vi "Initialize Hardware.vi"(7 "hardware config file":path, 8 "error in":errorcluster, 11 "device parameters":T2) -> (0 "error out":errorcluster, 3 "hardware handles":T1)   [LabVIEW 2020, in "Ballard MIL-STD-1553 Engine.lvlib" / "Custom Device.lvlib"]
uses:
  Custom Device.lvlib
  <instrlib>/BTICardLib/BTICardLV.lvlib
  <instrlib>/BTICardLib/Private/IO/Action-Status/Write External LED.vi
  <instrlib>/BTI1553Lib/BTI1553LV.lvlib
  Hardware Handles.ctl
  <instrlib>/BTI1553Lib/Private/Channel/Configure/Configure All From XML.vi
  <instrlib>/BTICardLib/Private/Initialize By Slot Number and Core Number.vi
  <instrlib>/BTICardLib/Private/Initialize By Card Number and Core Number.vi
  Shared/Device Parameters.ctl
  Shared/Initialization Method.ctl
panel:
  out "type string out":string
  out "product string out":string
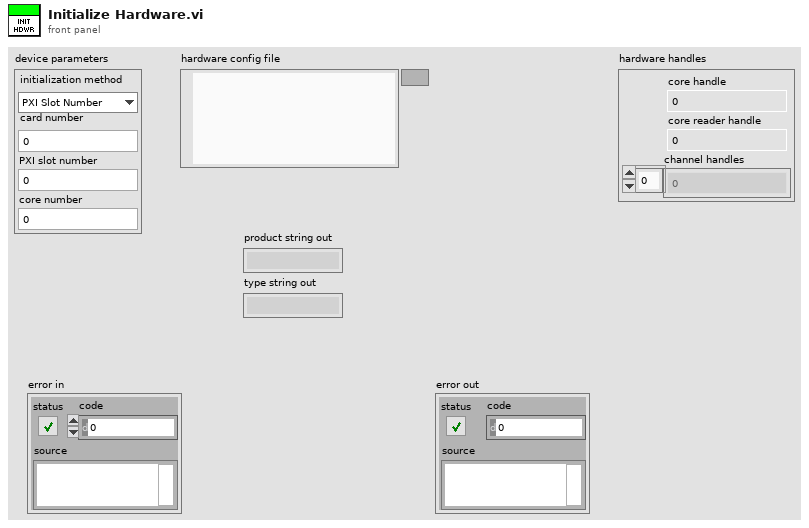
[diagram p1: front panel]
types:
  T1 = typedef "Ballard MIL-STD-1553 Engine.lvlib/Custom Device.lvlib/Hardware Handles.ctl" = cluster{"core handle":u64, "core reader handle":u64, "channel handles":u64[]}
  T2 = typedef "Device Parameters.ctl" = cluster{"initialization method":T3, "card number":i32, "PXI slot number":i32, "core number":i32}
  T3 = typedef "Initialization Method.ctl" = enum16{"PXI Slot Number", "Card Number"}
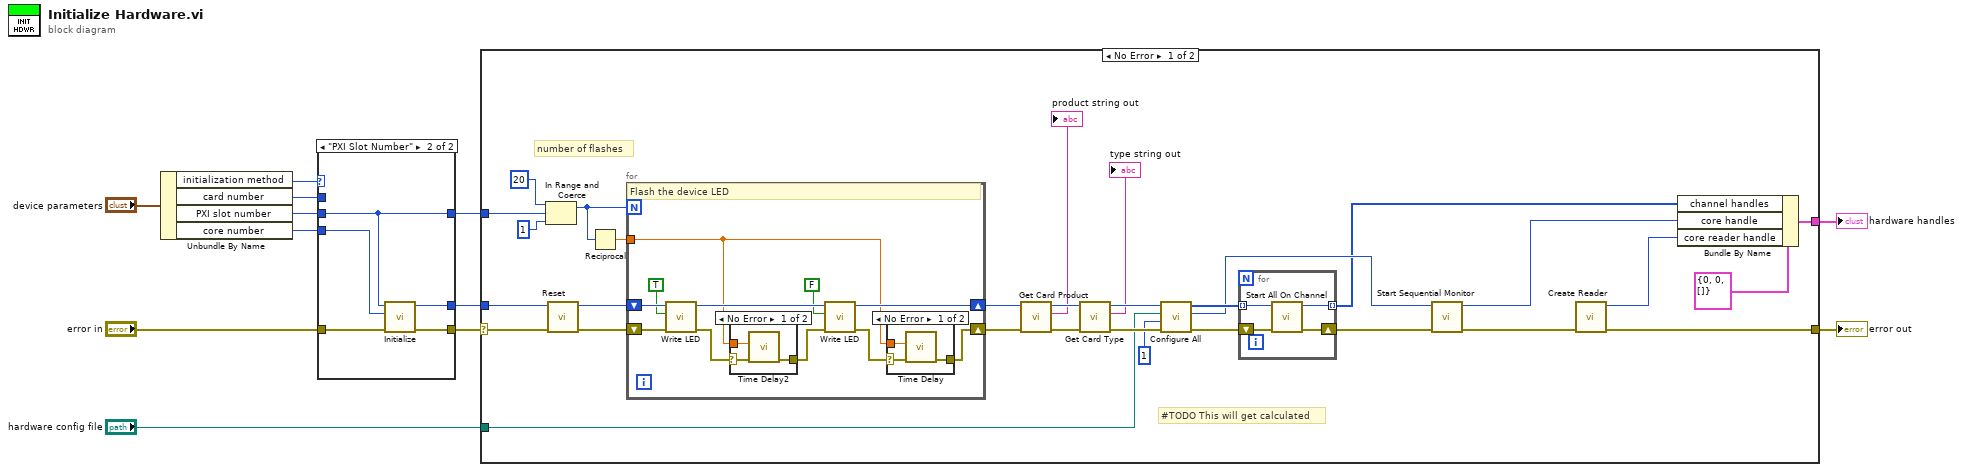
[diagram p0: block diagram]
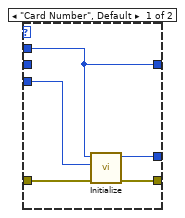
[diagram p5: hidden frame]
diagram:
  n1 = Unbundle By Name("device parameters") -> ("initialization method"=w5:T3, "card number"=w4:i32, "PXI slot number"=w8:i32, "core number"=w6:i32)
  n2 = case shown="\"PXI Slot Number\"" w5 {
    tunnel: [w17 w22] -> w3
    tunnel: [w16 w21] -> w1
    tunnel: w4 -> [w13 _]
    tunnel: "error in" -> [w15 w20]
    tunnel: w8 -> [_ w18]
    tunnel: w6 -> [w14 w19]
    tunnel: [w13 w18] -> w7
    frame "Card Number", Default {
      n3 = call-poly <instrlib>:"Initialize.vi"("error in (no error)"=w15, "core number"=w14, "card number"=w13) -> ("error out"=w16:errorcluster, "core handle out"=w17:u64)  [unwired: 7 in]
    }
    frame "PXI Slot Number" {
      n4 = call-poly <instrlib>:"Initialize.vi"("error in (no error)"=w20, "core number"=w19, "slot number"=w18) -> ("error out"=w21:errorcluster, "core handle out"=w22:u64)  [unwired: 7 in]
    }
  }
  n5 = case shown="No Error" w1 {
    selector: w1 -> [w45 w76]
    tunnel: w3 -> [w46 _]
    tunnel: w7 -> [w44 _]
    tunnel: "hardware config file" -> [w36 _]
    tunnel: [w35 w76] -> w10
    tunnel: [w23 _] -> w9
    frame No Error {
      # "#TODO This will get calculated"
      # "number of flashes"
      n6 = In Range and Coerce(upper limit=20 ("x"), x=w44, lower limit=1) -> (coerced(x)=w52:i32)  [unwired: 1 out]
      n7 = call <instrlib>:"Reset.vi"("error in (no error)"=w45, "core handle in"=w46) -> ("error out"=w47:errorcluster, "core handle out"=w48:u64)  [unwired: 8 in]
      n8 = Reciprocal(x=w52) -> (1/x=w51:dbl)
      n9 = for {
        N: w52 -> [_]
        shift-right: [w66] -> w38
        shift-left: w48 -> [w65]
        shift-right: [w60] -> w37
        shift-left: w47 -> [w64]
        tunnel: w51 -> [w57]
        # "Flash the device LED"
        n10 = call-poly <instrlib>:"Write LED.vi"("error in (no error)"=w64, "LED state"=TRUE, "core handle in"=w65) -> ("error out"=w59:errorcluster, "core handle out"=w67:u64)  [unwired: 7 in]
        n11 = case shown="No Error" w59 {
          selector: w59 -> [w70 w71]
          tunnel: [w69 w71] -> w58
          tunnel: w57 -> [w68 _]
          frame No Error {
            n12 = call "Time Delay2"("error in (no error)"=w70, "Delay Time (s)"=w68) -> ("error out"=w69:errorcluster)  [unwired: 9 in]
          }
          frame Error {
          }
        }
        n13 = call-poly <instrlib>:"Write LED.vi"("error in (no error)"=w58, "LED state"=FALSE, "core handle in"=w67) -> ("error out"=w61:errorcluster, "core handle out"=w66:u64)  [unwired: 7 in]
        n14 = case shown="No Error" w61 {
          selector: w61 -> [w74 w75]
          tunnel: [w73 w75] -> w60
          tunnel: w57 -> [w72 _]
          frame No Error {
            n15 = call "Time Delay"("error in (no error)"=w74, "Delay Time (s)"=w72) -> ("error out"=w73:errorcluster)  [unwired: 9 in]
          }
          frame Error {
          }
        }
      }
      n16 = call <instrlib>:"Get Card Product.vi"("error in (no error)"=w37, "core handle in"=w38) -> ("error out"=w40:errorcluster, "product string out"=→"product string out":string, "core handle out"=w39:u64)  [unwired: 7 in]
      n17 = call <instrlib>:"Get Card Type.vi"("error in (no error)"=w40, "core handle in"=w39) -> ("error out"=w43:errorcluster, "type string out"=→"type string out":string, "core handle out"=w42:u64)  [unwired: 7 in]
      n18 = call-poly <instrlib>:"Configure All.vi"("error in (no error)"=w43, "channel handle array size in"=1, "configuration file path"=w36, "core handle in"=w42) -> ("error out"=w30:errorcluster, "core handle out"=w28:u64, "channel handles out"=w31:u64[])  [unwired: 4 in, 1 out]
      n19 = for {
        tunnel: w31 -> [w56] mode=indexing
        tunnel: [w53] -> w24 mode=indexing
        shift-right: [w54] -> w29
        shift-left: w30 -> [w55]
        n20 = call <instrlib>:"Start All On Channel.vi"("error in (no error)"=w55, "channel handle in"=w56) -> ("error out"=w54:errorcluster, "channel handle out"=w53:u64)  [unwired: 8 in]
      }
      n21 = call <instrlib>:"Start Sequential Monitor.vi"("error in (no error)"=w29, "core handle in"=w28) -> ("error out"=w41:errorcluster, "core handle out"=w25:u64)  [unwired: 8 in]
      n22 = call <instrlib>:"Create Reader.vi"("error in (no error)"=w41) -> ("error out"=w35:errorcluster, "core reader handle out"=w26:u64)  [unwired: 9 in]
      n23 = Bundle By Name(cluster=T1 {"core handle"=0, "core reader handle"=0, "channel handles"=[]} ("hardware handles"), "channel handles"=w24, "core handle"=w25, "core reader handle"=w26) -> (w23:T1)
    }
    frame Error {
    }
  }
  "error out" <- w10
  "hardware handles" <- w9
